vi "1layer_Neuron.vi"(7 "Offset":dbl, 10 "Weight 1":dbl, 11 "Input 1":dbl) -> (4 "Output":dbl)   [LabVIEW 2016]
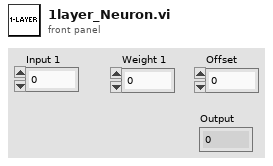
[diagram p1: front panel]
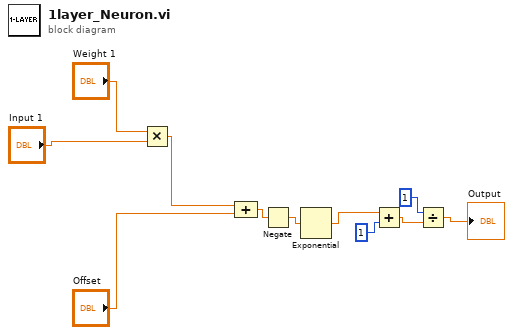
[diagram p0: block diagram]
diagram:
  n1 = Multiply(x="Weight 1", y="Input 1") -> (x*y=w10:dbl)
  n2 = Compound Arithmetic op=ADD(w10, "Offset") -> (w3:dbl)
  n3 = Negate(x=w3) -> (-x=w5:dbl)
  n4 = Exponential(1:w5) -> (0:w4:dbl)
  n5 = Add(x=w4, y=1) -> (x+y=w7:dbl)
  n6 = Divide(x=1, y=w7) -> (x/y=→"Output":dbl)
